vi "Do UI Action.vi"(8 "error in (no error)":errorcluster, 10 "UI Action":T1, 11 "Actor_UI_Template in":refnum<class "Actor_UI_Template.lvclass">) -> (0 "error out":errorcluster, 3 "Actor_UI_Template out":refnum<class "Actor_UI_Template.lvclass">)   [LabVIEW 2020, in "Actor_UI_Template.lvlib" / "Actor_UI_Template.lvclass"]
uses:
  Actor_UI_Template.lvclass
  UI Action Enum.ctl
  <vilib>/event_ctls.llb/usereventprio.ctl
  Actor_UI_Template.lvclass/Actor_UI_Template.ctl
  Actor_UI_Template.lvlib
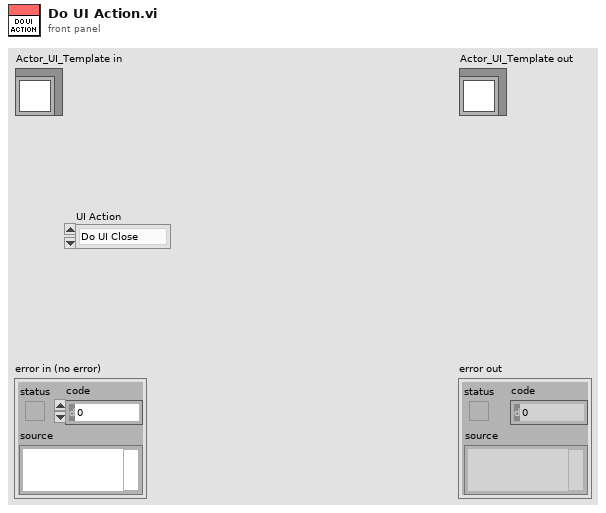
[diagram p1: front panel]
types:
  T1 = typedef "Actor_UI_Template.lvlib/UI Action Enum.ctl" = enum16{"Do UI Close"}
  T2 = typedef "usereventprio.ctl" = enum32{"high priority", "normal priority"}
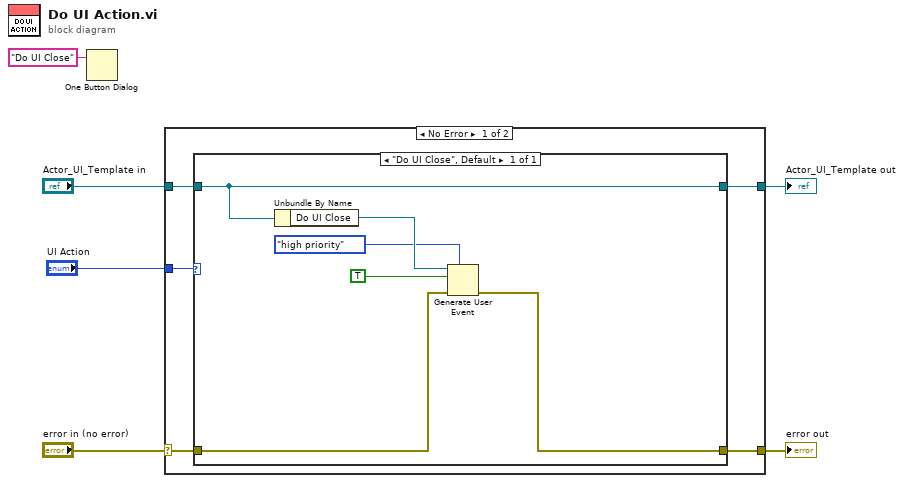
[diagram p0: block diagram]
diagram:
  n1 = One Button Dialog(message="Do UI Close") -> ()  [unwired: 1 in, 1 out]
  n2 = case shown="No Error" "error in (no error)" {
    selector: "error in (no error)" -> [w10 w19]
    tunnel: [w9 w19] -> w5
    tunnel: [w8 w18] -> w3
    tunnel: "Actor_UI_Template in" -> [w7 w18]
    tunnel: "UI Action" -> [w11 _]
    frame No Error {
      n3 = case shown="\"Do UI Close\", Default" w11 {
        tunnel: w10 -> [w13]
        tunnel: [w12] -> w9
        tunnel: [w17] -> w8
        tunnel: w7 -> [w17]
        frame "Do UI Close", Default {
          n4 = Unbundle By Name(w17) -> ("Do UI Close"=w16:refnum<user-event>)
          n5 = Generate User Event(priority (normal)=usereventprio."high priority", user event=w16, event data cluster=TRUE ("event data"), error in=w13) -> (error out=w12:errorcluster)  [unwired: 1 out]
        }
      }
    }
    frame Error {
    }
  }
  "error out" <- w5
  "Actor_UI_Template out" <- w3
